vi "NI VeriStand - Write Waveform(s).vi"   [LabVIEW 2020, in "NI_VS Custom Device Waveform API.lvlib"]
doc: "Writes an array of values to the waveform(s) associated with the specified write session. Use the Start Waveform(s) VI prior to this VI to set the waveform start time (t0) or start times. NI VeriStand considers all data this VI writes to be continuous unless the Start Waveform(s) VI executes again with a different start time."
uses:
  <vilib>/NI VeriStand/Custom Device Waveform API/NI_VS Custom Device Waveform API.lvlib
  <vilib>/NI VeriStand/Custom Device Waveform API/Multiple Waveforms Write (DBL)/Multiple Waveforms Write (DBL).lvclass
  <vilib>/NI VeriStand/Custom Device Waveform API/Single Waveform Write (DBL)/Single Waveform Write (DBL).lvclass
  <vilib>/NI VeriStand/Custom Device Waveform API/Single Waveform Write (CDB)/Single Waveform Write (CDB).lvclass
  <vilib>/NI VeriStand/Custom Device Waveform API/Multiple Waveforms Write (CDB)/Multiple Waveforms Write (CDB).lvclass
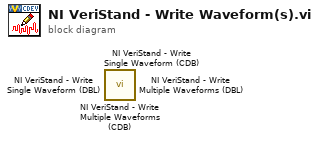
[diagram p0: block diagram]
diagram:
  n1 = call <vilib>:"NI VeriStand - Write Multiple Waveforms (CDB).vi"() -> ()  [unwired: 9 in, 3 out]
  n2 = call <vilib>:"NI VeriStand - Write Single Waveform (CDB).vi"() -> ()  [unwired: 9 in, 3 out]
  n3 = call <vilib>:"NI VeriStand - Write Single Waveform (DBL).vi"() -> ()  [unwired: 9 in, 3 out]
  n4 = call <vilib>:"NI VeriStand - Write Multiple Waveforms (DBL).vi"() -> ()  [unwired: 9 in, 3 out]
